vi "Main.vi"(8 "error in":errorcluster, 9 "Error Queue":refnum<queue>, 11 "Application Events":refnum<user-event>) -> (0 "error out":errorcluster)   [LabVIEW 2020, in "User Console.lvlib"]
doc: "VI Template with default error structure"
uses:
  User Console.lvlib
  Error/Controls/Error Message Object.ctl
  Controller/Controls/Application Modules.ctl
  Error/Controls/Error Commands.ctl
  Controller/Controls/Application Event Object.ctl
  Controller/Controls/Application Events.ctl
  Controls/Keypad.ctl
  Controls/Transactions.ctl
  Controls/Event Loop Data.ctl
  Controls/Operational Loop Data.ctl
  Controls/Operational Loop Commands.ctl
  Controller/Controller.lvlib
  Error/Error Handler.lvlib
panel:
  in  "Card Reader":bool
  in  "Transaction":T1
  in  "Keypad":T2
  # "[Covers: UI1]"
  # "[Covers: UI2]"
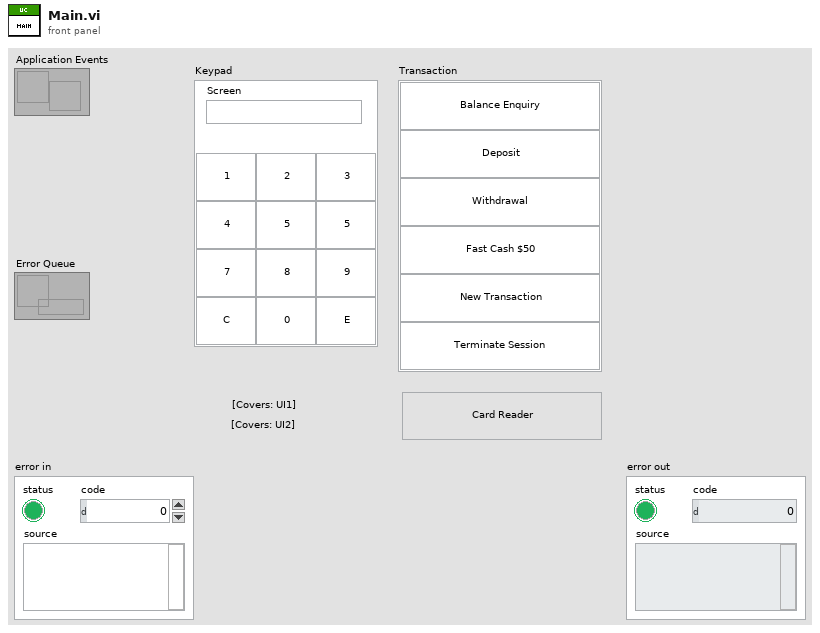
[diagram p1: front panel]
types:
  T1 = typedef "User Console.lvlib/Transactions.ctl" = cluster{"Balance Enquiry":bool, "Deposit":bool, "Withdrawal":bool, "Fast Cash $50":bool, "New Transaction":bool, "Terminate Session":bool}
  T2 = typedef "User Console.lvlib/Keypad.ctl" = cluster{"Key 1":bool, "Key 2":bool, "Key 3":bool, "Key 4":bool, "Key 5":bool, "Key 6":bool, "Key 7":bool, "Key 8":bool, "Key 9":bool, "Key C":bool, "Key 0":bool, "Key E":bool, "Screen":string}
  T3 = typedef "User Console.lvlib/Operational Loop Data.ctl" = cluster{"Current Module":T4}
  T4 = typedef "Controller.lvlib/Application Modules.ctl" = enum16{"Controller", "Error Module", "User Console", "Display Console", "Sensor Interface"}
  T5 = typedef "User Console.lvlib/Event Loop Data.ctl" = cluster{"Current Module":T4, "Timing":cluster{"isCounting":bool, "Timing Ticks Ms":i32, "Timing Target Sec":dbl, "Ticks Counter":i32}}
  T6 = typedef "Controller.lvlib/Application Events.ctl" = enum16{"Terminate App", "Initialize", "New Transaction", "Balance Inquiry", "Deposit", "Withdrawal", "Fast Cash 50$", "Terminate Session", "Login", "Verify Account"}
  T7 = typedef "User Console.lvlib/Operational Loop Commands.ctl" = enum16{"Shutdown"}
  T8 = enum16{"Load References", "Release References", "Get References"}
  T9 = typedef "Controller.lvlib/Controller Message Object.ctl" = cluster{"Commands":T10, "Source Module":T4, "Event Data":variant}
  T10 = typedef "Controller Commands.ctl" = enum16{"Shutdown"}
  T11 = typedef "Controller.lvlib/Application Event Object.ctl" = cluster{"Events":T6, "Source Module":T4, "Event Data":variant}
  T12 = cluster{"isCounting":bool, "Timing Ticks Ms":i32, "Timing Target Sec":dbl, "Ticks Counter":i32}
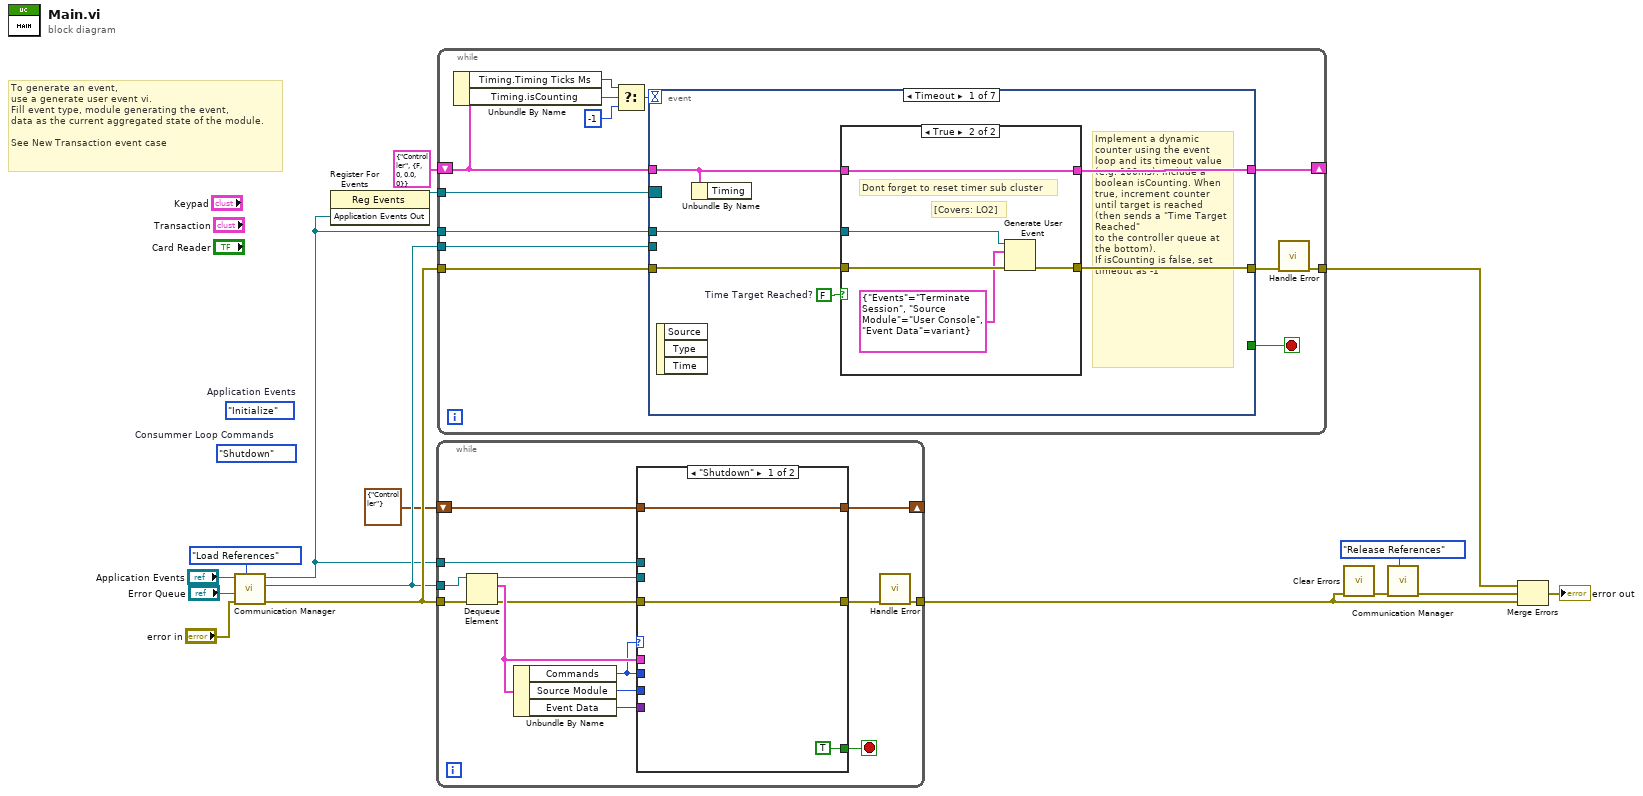
[diagram p0: block diagram]
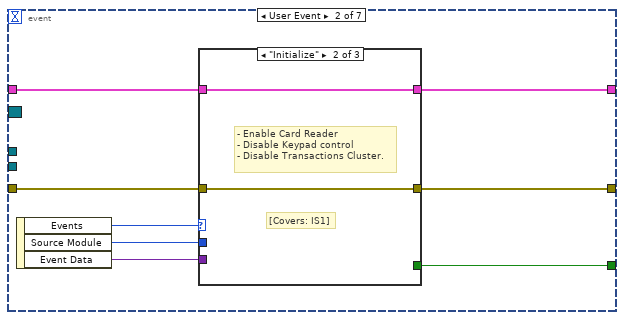
[diagram p4: hidden frame]
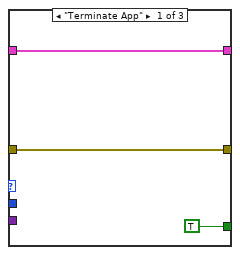
[diagram p5: hidden frame]
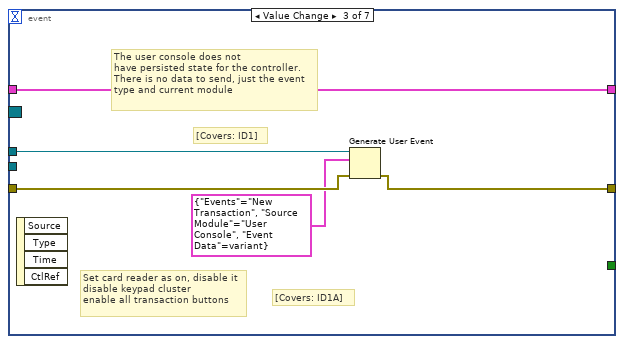
[diagram p7: hidden frame]
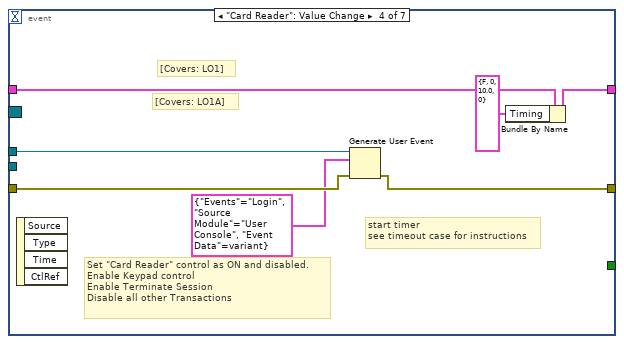
[diagram p8: hidden frame]
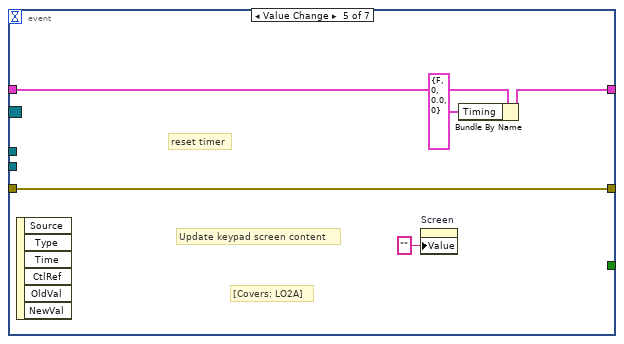
[diagram p9: hidden frame]
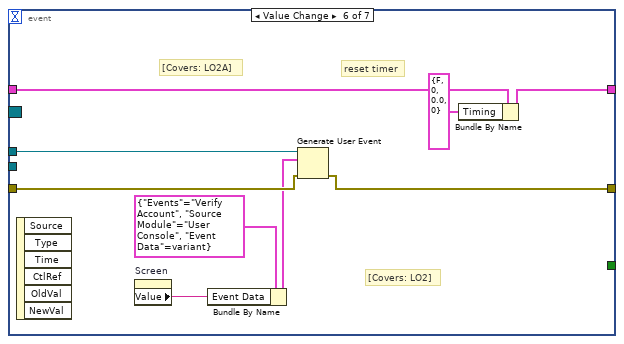
[diagram p10: hidden frame]
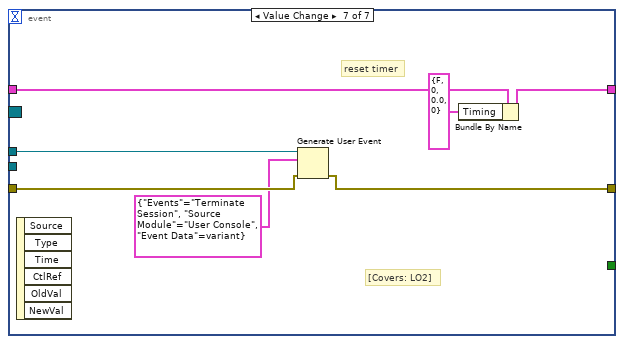
[diagram p11: hidden frame]
diagram:
  (unwired) Application_Events."Initialize"  # Application Events
  (unwired) Operational_Loop_Commands."Shutdown"  # Consummer Loop Commands
  # "To generate an event, \nuse a generate user event vi.\nFill event type, module generating the event,\ndata as the current aggregated state of the module.\n\nSee New Transaction event case"
  n1 = call "Communication Manager.vi"("Mode"=T8."Load References", "error in"="error in", "Error Queue"="Error Queue", "Application Events"="Application Events") -> ("error out"=w13:errorcluster, "Module Queue Out"=w5:refnum<queue>, "Application Events Out"=w4:refnum<user-event>)  [unwired: 4 in, 1 out]
  n2 = register-events(w4) -> (reference out=w3:refnum<event-registration>)  [unwired: 2 in, 1 out]
  n3 = while {
    tunnel: w13 -> [w29]
    tunnel: w5 -> [w28]
    tunnel: [w30] -> w7
    tunnel: w4 -> [w21]
    shift-right: [w18] -> _
    shift-left: T3 {"Current Module"=enum."Controller"} ("Operational Loop Data") -> [w19]
    stop <- w22 stop-if-true
    n4 = Dequeue Element(queue=w28, error in (no error)=w29) -> (queue out=w20:refnum<queue>, element=w26:T9, error out=w17:errorcluster)  [unwired: 1 in, 1 out]
    n5 = Unbundle By Name(w26) -> ("Commands"=w23:T10, "Source Module"=w25:T4, "Event Data"=w24:variant)
    n6 = case shown="\"Shutdown\"" w23 {
      tunnel: w17 -> [w33 w35]
      tunnel: [w33 w35] -> w27
      tunnel: w26 -> [_ _]
      tunnel: w23 -> [_ _]
      tunnel: w25 -> [_ _]
      tunnel: w24 -> [_ _]
      tunnel: [TRUE _] -> w22
      tunnel: w21 -> [_ _]
      tunnel: w20 -> [_ _]
      tunnel: w19 -> [w31 w34]
      tunnel: [w31 w34] -> w18
      frame "Shutdown" {
      }
      frame Default {
      }
    }
    n7 = call "Handle Error.vi"("error in"=w27) -> ("error out"=w30:errorcluster)  [unwired: 10 in]
  }
  n8 = while {
    tunnel: w13 -> [w47]
    tunnel: w4 -> [w46]
    tunnel: [w48] -> w11
    tunnel: w5 -> [w45]
    tunnel: w3 -> [w44]
    shift-right: [w41] -> _
    shift-left: T5 {"Current Module"=enum."Controller", "Timing"={"isCounting"=FALSE, "Timing Ticks Ms"=0, "Timing Target Sec"=0.0, "Ticks Counter"=0}} ("Event Loop Data") -> [w37]
    stop <- w42 stop-if-true
    n9 = Unbundle By Name(w37) -> ("Timing.Timing Ticks Ms"=w39:i32, "Timing.isCounting"=w40:bool)
    n10 = Select(t=w39, s=w40, f=-1) -> (s? t:f=w36:i32)
    n11 = event shown="[0] Timeout" {
      selector: w44 -> [_ _ _ _ _ _ _]
      dyn-events: _ -> [_ _ _ _ _ _ _]
      timeout: w36 -> [_ _ _ _ _ _ _]
      tunnel: w47 -> [w50 w68 w79 w87 w93 w98 w105]
      tunnel: w46 -> [w51 _ w80 w88 _ w99 w106]
      tunnel: w45 -> [_ _ _ _ _ _ _]
      tunnel: [w49 w69 w78 w86 w93 w97 w104] -> w43
      tunnel: [_ w64 _ _ _ _ _] -> w42
      tunnel: [w52 w63 w81 w83 w91 w101 w108] -> w41
      tunnel: w37 -> [w53 w62 w81 w84 w92 w102 w109]
      event Timeout {
        w54 = FALSE  # Time Target Reached?
        # "Implement a dynamic counter using the event\nloop and its timeout value (e.g. 100ms). Include a \nboolean isCounting. When true, increment counter\nuntil target is reached (then sends a \"Time Target Reached\"\nto the controller queue at the bottom).\nIf isCounting is false, set timeout as -1"
        n12 = event-data() -> ()  [unwired: 1 in, 3 out]
        n13 = Unbundle By Name(w53) -> ()  [unwired: 1 out]
        n14 = case shown="True" w54 {
          tunnel: w50 -> [w56 w60]
          tunnel: [w56 w59] -> w49
          tunnel: [w55 w61] -> w52
          tunnel: w53 -> [w55 w61]
          tunnel: w51 -> [_ w58]
          frame False {
          }
          frame True {
            # "[Covers: LO2]"
            # "Dont forget to reset timer sub cluster"
            n15 = Generate User Event(user event=w58, event data cluster=T11 {"Events"=enum."Terminate Session", "Source Module"=enum."User Console", "Event Data"=variant} ("event data"), error in=w60) -> (error out=w59:errorcluster)  [unwired: 1 in, 1 out]
          }
        }
      }
      event User Event {
        n16 = event-data() -> ("Events"=w67:T6, "Source Module"=w66:T4, "Event Data"=w65:variant)  [unwired: 1 in]
        n17 = case shown="\"Initialize\"" w67 {
          tunnel: [w72 w74 w76] -> w69
          tunnel: w68 -> [w72 w74 w76]
          tunnel: w66 -> [_ _ _]
          tunnel: w65 -> [_ _ _]
          tunnel: [TRUE _ _] -> w64
          tunnel: [w70 w73 w75] -> w63
          tunnel: w62 -> [w70 w73 w75]
          frame "Terminate App" {
          }
          frame "Initialize" {
            # "[Covers: IS1]"
            # "- Enable Card Reader \n- Disable Keypad control \n- Disable Transactions Cluster."
          }
          frame Default {
          }
        }
      }
      event Value Change {
        # "[Covers: ID1A]"
        # "[Covers: ID1]"
        # "Set card reader as on, disable it\ndisable keypad cluster\nenable all transaction buttons"
        # "The user console does not\nhave persisted state for the controller.\nThere is no data to send, just the event\ntype and current module"
        n18 = event-data() -> ()  [unwired: 1 in, 4 out]
        n19 = Generate User Event(user event=w80, event data cluster=T11 {"Events"=enum."New Transaction", "Source Module"=enum."User Console", "Event Data"=variant} ("event data"), error in=w79) -> (error out=w78:errorcluster)  [unwired: 1 in, 1 out]
      }
      event "Card Reader": Value Change {
        # "start timer\nsee timeout case for instructions"
        # "[Covers: LO1A]"
        # "Set \"Card Reader\" control as ON and disabled.\nEnable Keypad control\nEnable Terminate Session \nDisable all other Transactions"
        # "[Covers: LO1]"
        n20 = event-data() -> ()  [unwired: 1 in, 4 out]
        n21 = Generate User Event(user event=w88, event data cluster=T11 {"Events"=enum."Login", "Source Module"=enum."User Console", "Event Data"=variant} ("event data"), error in=w87) -> (error out=w86:errorcluster)  [unwired: 1 in, 1 out]
        n22 = Bundle By Name(cluster=w84, "Timing"=T12 {"isCounting"=FALSE, "Timing Ticks Ms"=0, "Timing Target Sec"=10.0, "Ticks Counter"=0}) -> (w83:T5)
      }
      event Value Change {
        # "[Covers: LO2A]"
        # "Update keypad screen content"
        # "reset timer"
        n23 = event-data() -> ()  [unwired: 1 in, 6 out]
        n24 = property on="Screen" class="Str"("Value"="") -> ()  [unwired: 2 in, 2 out]
        n25 = Bundle By Name(cluster=w92, "Timing"=T12 {"isCounting"=FALSE, "Timing Ticks Ms"=0, "Timing Target Sec"=0.0, "Ticks Counter"=0}) -> (w91:T5)
      }
      event Value Change {
        # "[Covers: LO2]"
        # "[Covers: LO2A]"
        # "reset timer"
        n26 = event-data() -> ()  [unwired: 1 in, 6 out]
        n27 = property on="Screen" class="Str"() -> ("Value"=w94:string)  [unwired: 2 in, 2 out]
        n28 = Bundle By Name(cluster=T11 {"Events"=enum."Verify Account", "Source Module"=enum."User Console", "Event Data"=variant} ("event data"), "Event Data"=w94) -> (w95:T11)
        n29 = Generate User Event(user event=w99, event data cluster=w95, error in=w98) -> (error out=w97:errorcluster)  [unwired: 1 in, 1 out]
        n30 = Bundle By Name(cluster=w102, "Timing"=T12 {"isCounting"=FALSE, "Timing Ticks Ms"=0, "Timing Target Sec"=0.0, "Ticks Counter"=0}) -> (w101:T5)
      }
      event Value Change {
        # "[Covers: LO2]"
        # "reset timer"
        n31 = event-data() -> ()  [unwired: 1 in, 6 out]
        n32 = Generate User Event(user event=w106, event data cluster=T11 {"Events"=enum."Terminate Session", "Source Module"=enum."User Console", "Event Data"=variant} ("event data"), error in=w105) -> (error out=w104:errorcluster)  [unwired: 1 in, 1 out]
        n33 = Bundle By Name(cluster=w109, "Timing"=T12 {"isCounting"=FALSE, "Timing Ticks Ms"=0, "Timing Target Sec"=0.0, "Ticks Counter"=0}) -> (w108:T5)
      }
    }
    n34 = call "Handle Error.vi"("error in"=w43) -> ("error out"=w48:errorcluster)  [unwired: 10 in]
  }
  n35 = call <vilib>:"Clear Errors.vi"("error in (no error)"=w7) -> ("error out"=w10:errorcluster)  [unwired: 5 in, 1 out]
  n36 = call "Communication Manager.vi"("Mode"=T8."Release References", "error in"=w10) -> ("error out"=w6:errorcluster)  [unwired: 6 in, 3 out]
  n37 = Merge Errors(w11, w6, w7) -> (→"error out":errorcluster)
